vi "Main.vi"(8 "error in (no error)":errorcluster, 11 "Dispatcher in":refnum<class "Dispatcher Thread.lvclass">) -> (0 "error out":errorcluster, 3 "Dispatcher out":refnum<class "Dispatcher Thread.lvclass">)   [LabVIEW 2017, in "DSF Core.lvlib" / "Dispatcher Thread.lvclass"]
uses:
  Dispatcher Thread.lvclass
  C:/Git/DSF/Data Sharing Framework/Source/Core/Engine/Classes/Thread/Thread.lvclass
  Thread/Thread.lvclass
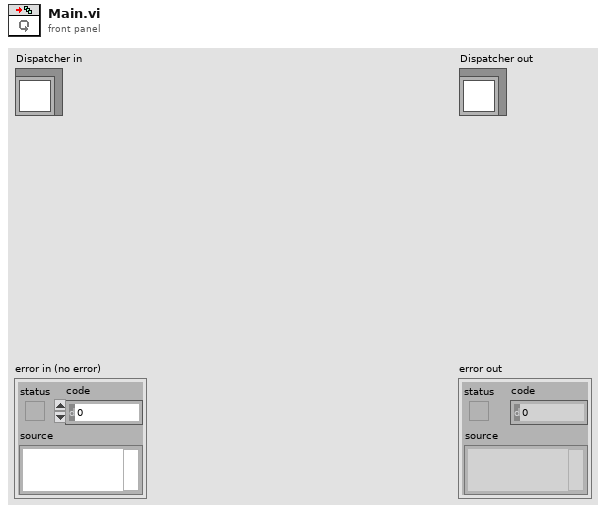
[diagram p1: front panel]
types:
  T1 = typedef "DSF Core.lvlib/Dispatcher Interface.lvclass/Command Data.ctl" = cluster{"Command":T2, "Parameters":T3}
  T2 = typedef "DSF Core.lvlib/Dispatcher Interface.lvclass/Command.ctl" = enum8{"Rx", "Tx", "Set Inline Buffer", "Shutdown"}
  T3 = typedef "DSF Core.lvlib/Dispatcher Interface.lvclass/Parameters.ctl" = cluster{"arg1":u64, "arg2":u64}
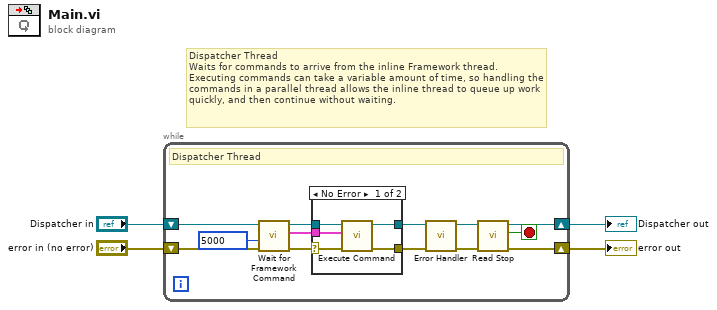
[diagram p0: block diagram]
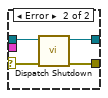
[diagram p2: hidden frame]
diagram:
  # "Dispatcher Thread\nWaits for commands to arrive from the inline Framework thread. Executing commands can take a variable amount of time, so handling the commands in a parallel thread allows the inline thread to queue up work quickly, and then continue without waiting."
  n1 = while {
    shift-right: [w12] -> w4
    shift-left: "error in (no error)" -> [w9]
    shift-right: [w13] -> w3
    shift-left: "Dispatcher in" -> [w5]
    stop <- w11 stop-if-true
    # "Dispatcher Thread"
    n2 = call "Wait for Framework Command.vi"("error in (no error)"=w9, "timeout in ms (5000)"=5000 ("timeout in ms (0)"), "Dispatcher in"=w5) -> ("error out"=w7:errorcluster, "command"=w6:T1, "Dispatcher out"=w8:refnum<class "Dispatcher Thread.lvclass">)  [unwired: 6 in]
    n3 = case shown="No Error" w7 {
      selector: w7 -> [w18 w23]
      tunnel: [w22 w25] -> w17
      tunnel: [w21 w24] -> w16
      tunnel: w8 -> [w20 w26]
      tunnel: w6 -> [w19 _]
      frame No Error {
        n4 = call "Execute Command.vi"("error in (no error)"=w18, "command"=w19, "Dispatcher in"=w20) -> ("error out"=w21:errorcluster, "Dispatcher out"=w22:refnum<class "Dispatcher Thread.lvclass">)  [unwired: 7 in]
      }
      frame Error {
        n5 = call "Dispatch Shutdown.vi"("error in (no error)"=w23, "Dispatcher in"=w26) -> ("error out"=w24:errorcluster, "Dispatcher out"=w25:refnum<class "Dispatcher Thread.lvclass">)  [unwired: 8 in]
      }
    }
    n6 = call "Error Handler.vi"("error in (no error)"=w16, "Dispatcher in"=w17) -> ("error out"=w14:errorcluster, "Dispatcher out"=w15:refnum<class "Dispatcher Thread.lvclass">)  [unwired: 8 in]
    n7 = call "Read Stop.vi"("error in (no error)"=w14, "Thread in"=w15) -> ("error out"=w12:errorcluster, "stop"=w11:bool, "Thread out"=w13:refnum<class "Dispatcher Thread.lvclass">)  [unwired: 7 in]
  }
  "error out" <- w4
  "Dispatcher out" <- w3
